vi "Read Waveform Data.vi"(8 "error in (no error)":errorcluster, 10 "Timeout (10000 ms)":i32=10000 min=1, 11 "VISA resource name":refnum<visa-resource-name>) -> (0 "error out":errorcluster, 2 "Waveform Data":string, 3 "VISA resource name out":refnum<visa-resource-name>)   [LabVIEW 2021, in "Yokogawa WT1800 Series.lvlib"]
doc: "Queries the waveform data from the instruments."
uses:
  <instrlib>/Yokogawa WT1800 Series/Yokogawa WT1800 Series.lvlib
panel:
  # "ms"
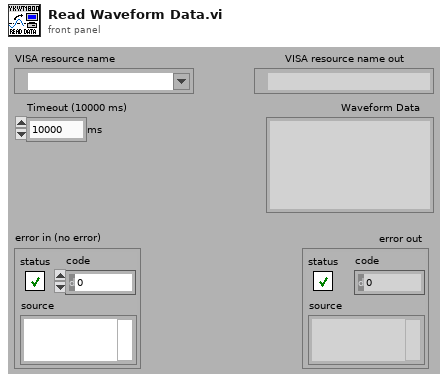
[diagram p1: front panel]
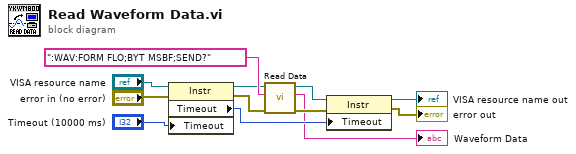
[diagram p0: block diagram]
diagram:
  n1 = property on="プロパティノード" class="Instr"(reference="VISA resource name", error in="error in (no error)", "Timeout"="Timeout (10000 ms)") -> (reference out=w5:refnum<visa-resource-name>, error out=w4:errorcluster, "Timeout"=w12:u32)
  n2 = call <instrlib>:"Read Data.vi"("error in (no error)"=w4, "Send Command (Empty)"=":WAV:FORM FLO;BYT MSBF;SEND?", "VISA resource name"=w5) -> ("error out"=w2:errorcluster, "Read Data"=→"Waveform Data":string, "VISA resource name out"=w3:refnum<visa-resource-name>)  [unwired: 5 in, 1 out]
  n3 = property on="プロパティノード" class="Instr"(reference=w3, error in=w2, "Timeout"=w12) -> (reference out=→"VISA resource name out":refnum<visa-resource-name>, error out=→"error out":errorcluster)
